vi "DropPolicyString.vi"(8 "error in (no error)":errorcluster, 11 "DropPolicy":T1) -> (0 "error out":errorcluster, 3 "DropPolicyString":string)   [LabVIEW 2026, in "Lumberjack.lvlib"]
doc: "Converts a DropPolicy enum to its member-name string (DropOldest, DropNewest, LevelAware).\nUsed to build the config DTO; round-trip partner of DropPolicyFromString. Pure; no state, no I/O.\nLumberjack.lvlib, community (friend of Tests.lvlib)."
uses:
  Lumberjack.lvlib
  TypeDefs/DropPolicy.ctl
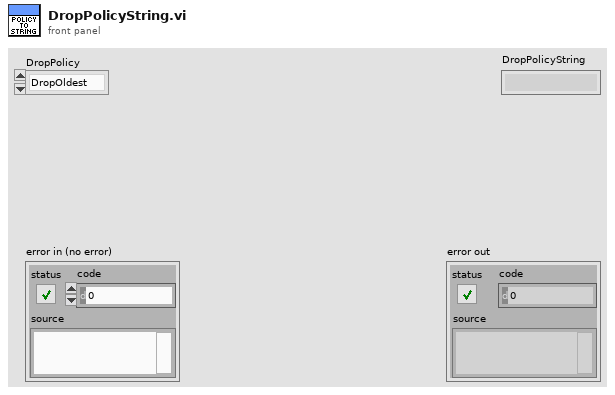
[diagram p1: front panel]
types:
  T1 = typedef "Lumberjack.lvlib/DropPolicy.ctl" = enum16{"DropOldest", "DropNewest", "LevelAware"}
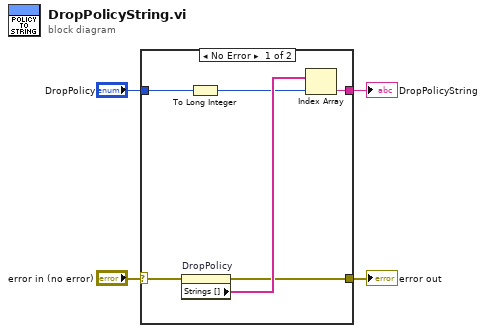
[diagram p0: block diagram]
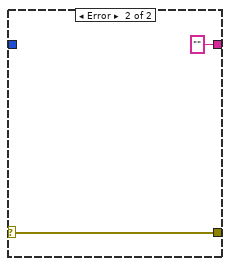
[diagram p2: hidden frame]
diagram:
  n1 = case shown="No Error" "error in (no error)" {
    selector: "error in (no error)" -> [w5 w12]
    tunnel: [w8 ""] -> w4
    tunnel: [w7 w12] -> w3
    tunnel: "DropPolicy" -> [w6 _]
    frame No Error {
      n2 = property on="DropPolicy" class="Enum (strict)"(error in=w5) -> (error out=w7:errorcluster, "Strings []"=w10:string[])  [unwired: 1 in, 1 out]
      n3 = To Long Integer(number=w6) -> (32bit integer=w9:i32)
      n4 = Index Array(array=w10, index=w9) -> (element=w8:string)
    }
    frame Error {
    }
  }
  "error out" <- w3
  "DropPolicyString" <- w4
